vi "MeasurementFinished.vi"(8 "error in (no error)":errorcluster, 10 "Error":bool, 11 "SPIController in":refnum<class "SPIController.lvclass">) -> (0 "error out":errorcluster, 3 "SPIController out":refnum<class "SPIController.lvclass">)   [LabVIEW 2023, in "SPIController.lvlib" / "SPIController.lvclass"]
uses:
  SPIController.lvclass
  SPIController.lvclass/SPIController.ctl
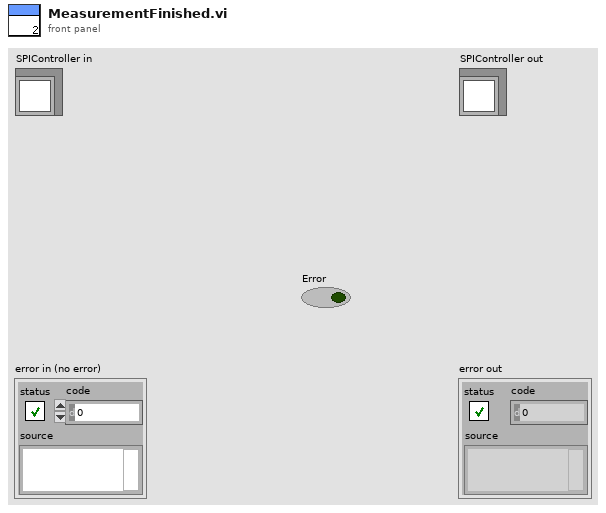
[diagram p1: front panel]
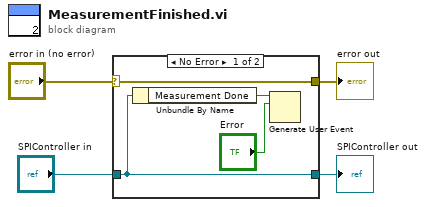
[diagram p0: block diagram]
diagram:
  n1 = case shown="No Error" "error in (no error)" {
    selector: "error in (no error)" -> [w8 w10]
    tunnel: [w8 w10] -> w3
    tunnel: [w7 w9] -> w1
    tunnel: "SPIController in" -> [w7 w9]
    frame No Error {
      n2 = Unbundle By Name(w7) -> ("Measurement Done"=w6:refnum<user-event>)
      n3 = Generate User Event(user event=w6, event data cluster="Error") -> ()  [unwired: 2 in, 2 out]
    }
    frame Error {
    }
  }
  "error out" <- w3
  "SPIController out" <- w1
